vi "Globalvariable.vi"() -> ()   [LabVIEW 2012]
panel:
  in  "String":string
  in  "Account":dbl
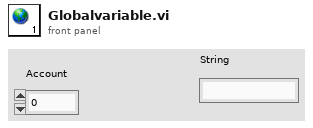
[diagram p1: front panel]
diagram:
